vi "Update Item Overlay.vi"(7 "Check overlay?":bool, 8 "error in (no error)":errorcluster, 9 "Status":i32, 10 "Item":T1) -> (0 "error out":errorcluster)   [LabVIEW 2020, in "Icon Decorator.lvlib" / "Icon Decorator.lvclass"]
doc: "Refresh the overlay for the Test Case class."
uses:
  Icon Decorator.lvclass
  <resource>/Framework/Providers/API/ItemRef.ctl
  <resource>/Framework/Providers/API/mxLvUpdateUI.ctl
  <resource>/Framework/Providers/API/mxLvOverlayState.ctl
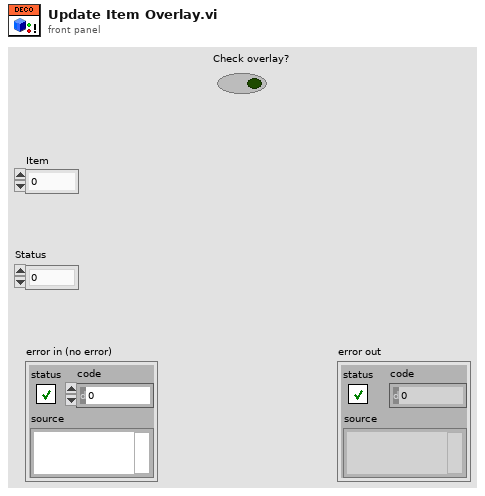
[diagram p1: front panel]
types:
  T1 = typedef "ItemRef.ctl" = u64
  T2 = typedef "mxLvUpdateUI.ctl" = cluster{"Action":u32, "Optional param 1":string, "Optional param 2":i32, "Optional param 3":string}
  T3 = typedef "mxLvOverlayState.ctl" = cluster{"Overlay Alias":string, "Active":bool}
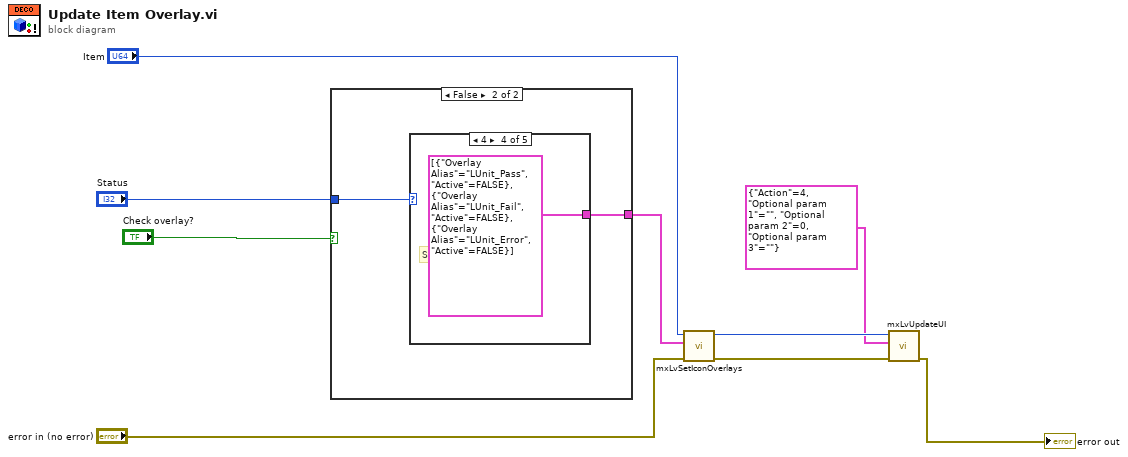
[diagram p0: block diagram]
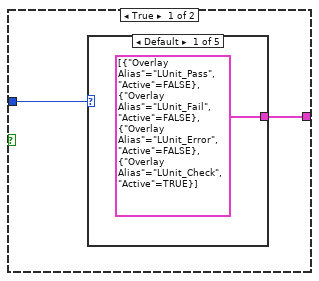
[diagram p2: hidden frame]
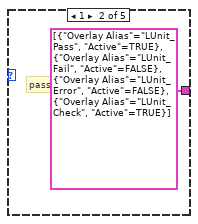
[diagram p3: hidden frame]
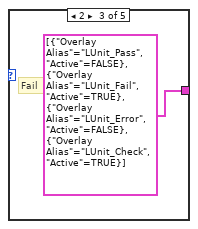
[diagram p4: hidden frame]
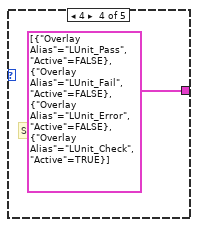
[diagram p5: hidden frame]
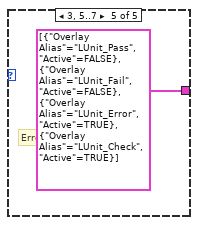
[diagram p6: hidden frame]
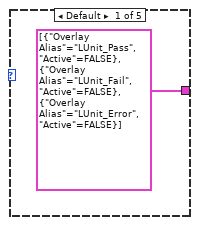
[diagram p7: hidden frame]
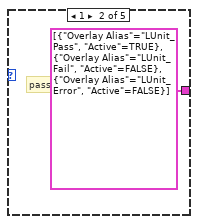
[diagram p8: hidden frame]
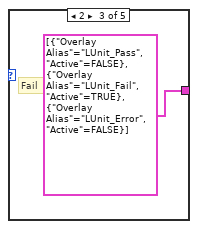
[diagram p9: hidden frame]
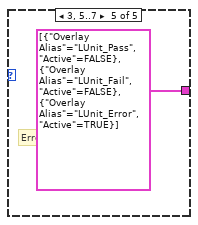
[diagram p10: hidden frame]
diagram:
  n1 = case shown="False" "Check overlay?" {
    tunnel: "Status" -> [w11 w18]
    tunnel: [w10 w17] -> w2
    frame True {
      n2 = case shown="Default" w11 {
        tunnel: [T3[] [{"Overlay Alias"="LUnit_Pass", "Active"=FALSE}, {"Overlay Alias"="LUnit_Fail", "Active"=FALSE}, {"Overlay Alias"="LUnit_Error", "Active"=FALSE}, {"Overlay Alias"="LUnit_Check", "Active"=TRUE}] ("Array") T3[] [{"Overlay Alias"="LUnit_Pass", "Active"=TRUE}, {"Overlay Alias"="LUnit_Fail", "Active"=FALSE}, {"Overlay Alias"="LUnit_Error", "Active"=FALSE}, {"Overlay Alias"="LUnit_Check", "Active"=TRUE}] ("Array") T3[] [{"Overlay Alias"="LUnit_Pass", "Active"=FALSE}, {"Overlay Alias"="LUnit_Fail", "Active"=TRUE}, {"Overlay Alias"="LUnit_Error", "Active"=FALSE}, {"Overlay Alias"="LUnit_Check", "Active"=TRUE}] ("Array") T3[] [{"Overlay Alias"="LUnit_Pass", "Active"=FALSE}, {"Overlay Alias"="LUnit_Fail", "Active"=FALSE}, {"Overlay Alias"="LUnit_Error", "Active"=FALSE}, {"Overlay Alias"="LUnit_Check", "Active"=TRUE}] ("Array") T3[] [{"Overlay Alias"="LUnit_Pass", "Active"=FALSE}, {"Overlay Alias"="LUnit_Fail", "Active"=FALSE}, {"Overlay Alias"="LUnit_Error", "Active"=TRUE}, {"Overlay Alias"="LUnit_Check", "Active"=TRUE}] ("Array")] -> w10
        frame Default {
        }
        frame 1 {
          # "pass"
        }
        frame 2 {
          # "Fail"
        }
        frame 4 {
          # "Skip"
        }
        frame 3, 5..7 {
          # "Error"
        }
      }
    }
    frame False {
      n3 = case shown="4" w18 {
        tunnel: [T3[] [{"Overlay Alias"="LUnit_Pass", "Active"=FALSE}, {"Overlay Alias"="LUnit_Fail", "Active"=FALSE}, {"Overlay Alias"="LUnit_Error", "Active"=FALSE}] ("Array") T3[] [{"Overlay Alias"="LUnit_Pass", "Active"=TRUE}, {"Overlay Alias"="LUnit_Fail", "Active"=FALSE}, {"Overlay Alias"="LUnit_Error", "Active"=FALSE}] ("Array") T3[] [{"Overlay Alias"="LUnit_Pass", "Active"=FALSE}, {"Overlay Alias"="LUnit_Fail", "Active"=TRUE}, {"Overlay Alias"="LUnit_Error", "Active"=FALSE}] ("Array") T3[] [{"Overlay Alias"="LUnit_Pass", "Active"=FALSE}, {"Overlay Alias"="LUnit_Fail", "Active"=FALSE}, {"Overlay Alias"="LUnit_Error", "Active"=FALSE}] ("Array") T3[] [{"Overlay Alias"="LUnit_Pass", "Active"=FALSE}, {"Overlay Alias"="LUnit_Fail", "Active"=FALSE}, {"Overlay Alias"="LUnit_Error", "Active"=TRUE}] ("Array")] -> w17
        frame Default {
        }
        frame 1 {
          # "pass"
        }
        frame 2 {
          # "Fail"
        }
        frame 4 {
          # "Skip"
        }
        frame 3, 5..7 {
          # "Error"
        }
      }
    }
  }
  n4 = call <resource>:"mxLvSetIconOverlays.vi"("error in"="error in (no error)", "Overlay States"=w2, "Item"="Item") -> ("error out"=w6:errorcluster, "Item"=w5:T1)  [unwired: 7 in]
  n5 = call <resource>:"mxLvUpdateUI.vi"("error in"=w6, "Update UI Settings"=T2 {"Action"=4, "Optional param 1"="", "Optional param 2"=0, "Optional param 3"=""}, "Item"=w5) -> ("error out"=→"error out":errorcluster)  [unwired: 7 in, 1 out]
